vi "Write SampleClock.vi"(8 "error in (no error)":errorcluster, 10 "SampleClock":T1 {"sample mode" items=["Finite Samples"=10178, "Continuous Samples"=10123, "Hardware Timed Single Point"=12522]; "TimebaseRate" format="%#_6p"}, 11 "NiDaqMx in":refnum<class "NiDaqMx.lvclass">) -> (0 "error out":errorcluster, 3 "NiDaqMx out":refnum<class "NiDaqMx.lvclass">)   [LabVIEW 2014, in "DigitizerPlugins.lvlib" / "NiDaqMx.lvclass"]
uses:
  NiDaqMx.lvclass
  SampleClock.ctl
  NiDaqMx.lvclass/NiDaqMx.ctl
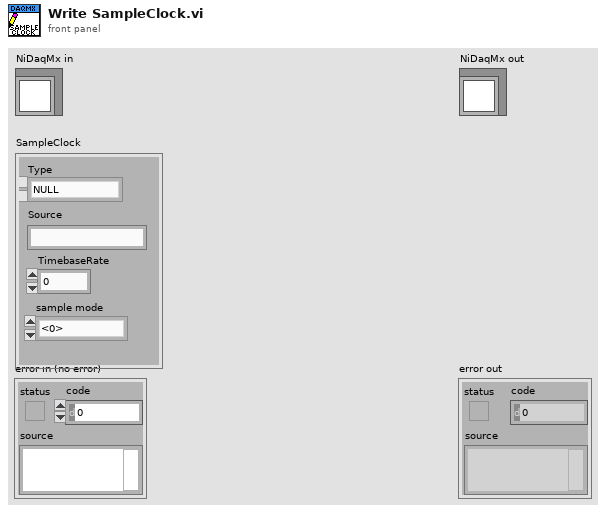
[diagram p1: front panel]
types:
  T1 = typedef "DigitizerPlugins.lvlib/NiDaqMx.lvclass/SampleClock.ctl" = cluster{"Type":enum16{"NULL", "Onboard", "External", "Software", "Interval"}, "Source":string, "TimebaseRate":dbl, "sample mode":i32}
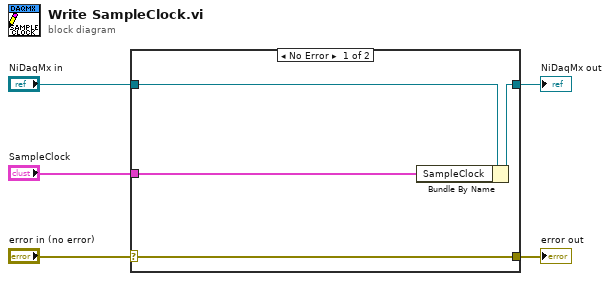
[diagram p0: block diagram]
diagram:
  n1 = case shown="No Error" "error in (no error)" {
    selector: "error in (no error)" -> [w9 w10]
    tunnel: [w9 w10] -> w4
    tunnel: [w7 w11] -> w2
    tunnel: "NiDaqMx in" -> [w8 w11]
    tunnel: "SampleClock" -> [w6 _]
    frame No Error {
      n2 = Bundle By Name(cluster=w8, "SampleClock"=w6) -> (w7:refnum<class "NiDaqMx.lvclass">)
    }
    frame Error {
    }
  }
  "error out" <- w4
  "NiDaqMx out" <- w2
